vi "Ramsete_Execute_PackTuning.vi"(5 "B":dbl=2.0, 6 "Heading Tolerance RAD":dbl=0.035, 7 "Zeta":dbl=0.7, 8 "Y Tolerance M":dbl=0.051, 9 "X Tolerance M":dbl=0.051, 10 "Max Speed M/S":dbl, 11 "Track Width M":dbl) -> (3 "RAMSETE_EXE_TUNING":T1={"B"=2.0, "Zeta"=0.7, "X Tolerance M"=2.0, "Y Tolerance M"=0.7, "Heading Tolerance RAD"=0.7, "Track Width M"=2.0, "Max Speed M/S"=2.0} {"Max Speed M/S" format="%13.4f"; "Track Width M" format="%13.4f"; "Heading Tolerance RAD" format="%13.4f"; "Y Tolerance M" format="%13.4f"; "X Tolerance M" format="%13.4f"; "Zeta" format="%13.4f"; "B" format="%13.4f"})   [LabVIEW 2019, in "Trajectory_Library.lvlib"]
doc: "Packs tuning parameters for the Ramsete EXE VI (Which is designed for a differential drive robot)\n\nInputs:\n - b - Tuning parameter (b > 0), radians^2 / meters^2, for which larger values make convergence more aggressive like a proportional term. (Default 2.0)\n - zeta - Tuning parameter (0 <; zeta < 1), / radians, for which larger values provide more damping in response. (Default 07 )\n - track width -- distance between right and left wheels on a differential drive robot (Meters)\n - Max Speed -- The maximum wheel speed (Meters/Second)\n - X Tolerance -- The desired allowable X position deviation (Meters). This is only used to calculate At Reference. (Default 0.051)\n - Y Tolerance -- The desired allowable Y position deviation (Meters). This is only used to calculate At Reference. (Default 0.051)\n - Heading Tolerance -- The desired allowable rotation deviation (Radians). This is only used to calculate At Reference. (Default 0.035)\n\nOutputs:\n - Ramseete EXE tuning -- Data cluster to be used as input to the Ramsete EXE VI."
uses:
  Trajectory_Library.lvlib
  RAMSETE_EXE_TUNING.ctl
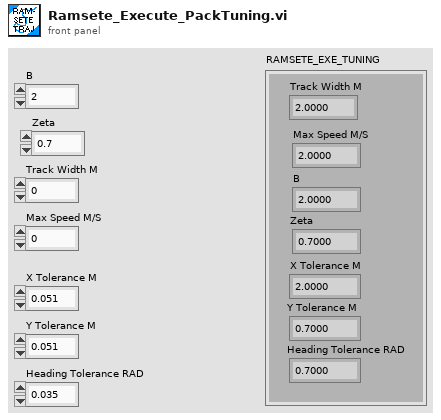
[diagram p1: front panel]
types:
  T1 = typedef "Trajectory_Library.lvlib/RAMSETE_EXE_TUNING.ctl" = cluster{"B":dbl, "Zeta":dbl, "X Tolerance M":dbl, "Y Tolerance M":dbl, "Heading Tolerance RAD":dbl, "Track Width M":dbl, "Max Speed M/S":dbl}
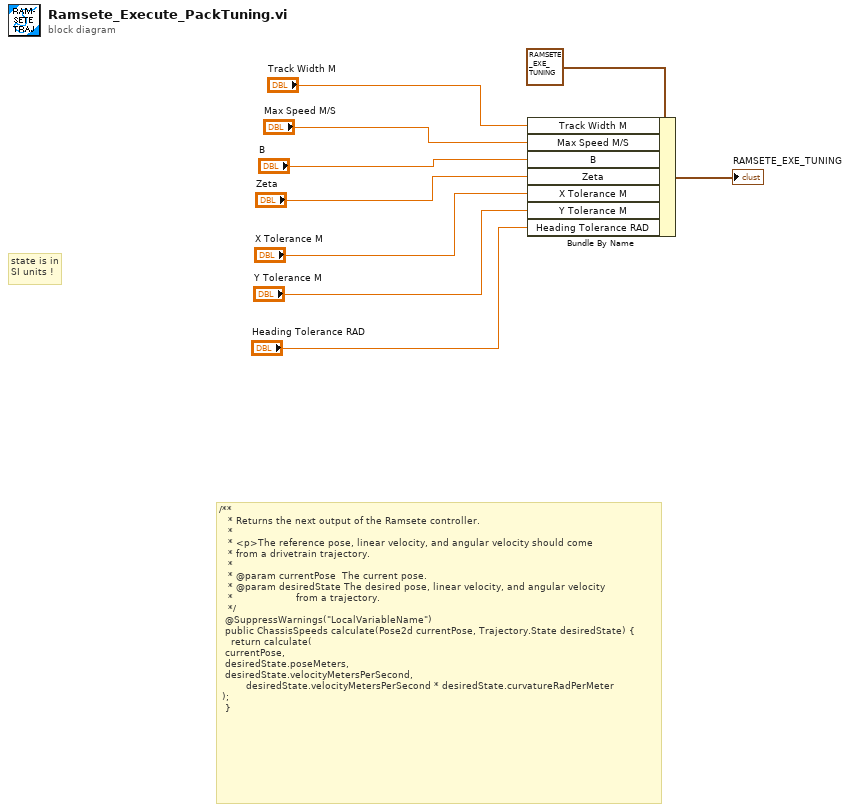
[diagram p0: block diagram]
diagram:
  # "state is in\nSI units !"
  # "/**\n   * Returns the next output of the Ramsete controller.\n   *\n   * <p>The reference pose, linear velocity, and angular velocity should come\n   * from a drivetrain trajectory.\n   *\n   * @param currentPose  The current pose.\n   * @param desiredState The desired pose, linear velocity, and angular velocity\n   *                     from a trajectory.\n   */\n  @SuppressWarnings(\"LocalVariableName\")\n  public ChassisSpeeds calculate(Pose2d currentPose, Trajectory.State desiredState) {\n    return calculate(\n\t\tcurrentPose, \n\t\tdesiredState.poseMeters, \n\t\tdesiredState.velocityMetersPerSecond,\n        \tdesiredState.velocityMetersPerSecond * desiredState.curvatureRadPerMeter\n\t);\n  }"
  n1 = Bundle By Name(cluster=T1 {"B"=2.0, "Zeta"=0.7, "X Tolerance M"=0.051, "Y Tolerance M"=0.051, "Heading Tolerance RAD"=0.035, "Track Width M"=2.0, "Max Speed M/S"=2.0} ("RAMSETE_EXE_TUNING"), "Track Width M"="Track Width M", "Max Speed M/S"="Max Speed M/S", "B"="B", "Zeta"="Zeta", "X Tolerance M"="X Tolerance M", "Y Tolerance M"="Y Tolerance M", "Heading Tolerance RAD"="Heading Tolerance RAD") -> (→"RAMSETE_EXE_TUNING":T1)
